vi "VNAfreq.vi"(1 "Center Freq (Hz)":dbl, 2 "Span Freq (Hz)":dbl, 3 "Sweep Points":i32) -> (0 "VNA Freq":dbl[](array[numeric]))   [LabVIEW 2017]
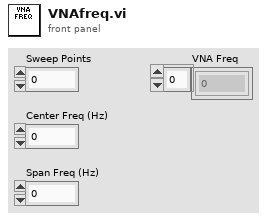
[diagram p1: front panel]
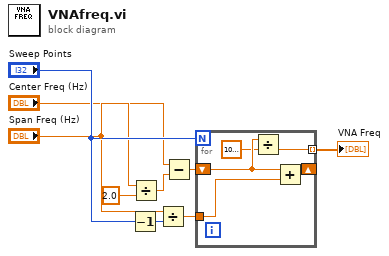
[diagram p0: block diagram]
diagram:
  n1 = Decrement(x="Sweep Points") -> (x-1=w4:i32)
  n2 = Divide(x="Span Freq (Hz)", y=2.0) -> (x/y=w2:dbl)
  n3 = Divide(x="Span Freq (Hz)", y=w4) -> (x/y=w5:dbl)
  n4 = Subtract(x="Center Freq (Hz)", y=w2) -> (x-y=w3:dbl)
  n5 = for {
    N: "Sweep Points" -> [_]
    shift-right: [w14] -> _
    shift-left: w3 -> [w11]
    tunnel: [w12] -> w9 mode=indexing
    tunnel: w5 -> [w13]
    n6 = Divide(x=w11, y=1000000000.0 ("x")) -> (x/y=w12:dbl)
    n7 = Add(x=w11, y=w13) -> (x+y=w14:dbl)
  }
  "VNA Freq" <- w9
